vi "add_virtual_folder.vi"(8 "error in":errorcluster, 10 "Name":string="type definitions", 11 "folder reference in":refnum<vi>) -> (0 "error out":errorcluster, 3 "folder reference out":refnum<vi>)   [LabVIEW 2010]
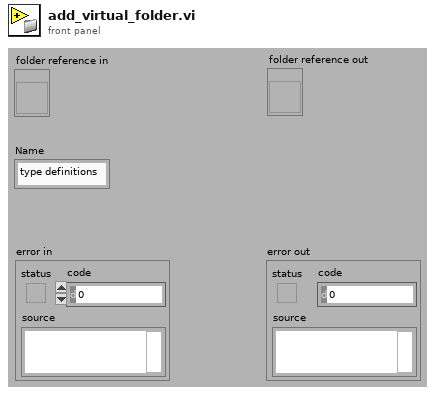
[diagram p1: front panel]
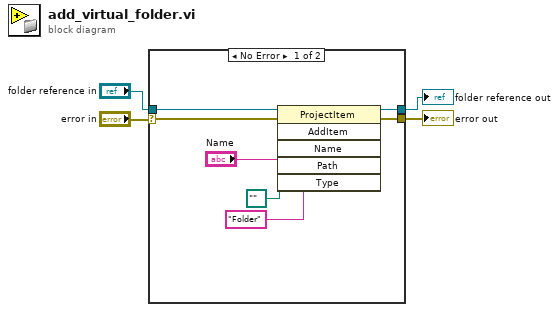
[diagram p0: block diagram]
diagram:
  n1 = case shown="No Error" "error in" {
    selector: "error in" -> [w5 w13]
    tunnel: "folder reference in" -> [w11 w12]
    tunnel: [w10 w12] -> w3
    tunnel: [w6 w13] -> w2
    frame No Error {
      n2 = invoke class="ProjectItem" method="AddItem"(reference=w11, error in=w5, "Name"="Name", "Path"=path "", "Type"="Folder") -> (reference out=w10:refnum<vi>, error out=w6:errorcluster)  [unwired: 1 in, 4 out]
    }
    frame Error {
    }
  }
  "folder reference out" <- w3
  "error out" <- w2
